vi "CTRE_Phoenix_CANcoder_GetPolymorphic.vi"   [LabVIEW 2020]
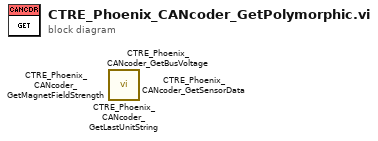
[diagram p0: block diagram]
diagram:
  n1 = call <vilib>:"CTRE_Phoenix_CANcoder_GetLastUnitString.vi"() -> ()  [unwired: 13 in, 3 out]
  n2 = call <vilib>:"CTRE_Phoenix_CANcoder_GetBusVoltage.vi"() -> ()  [unwired: 13 in, 3 out]
  n3 = call <vilib>:"CTRE_Phoenix_CANcoder_GetMagnetFieldStrength.vi"() -> ()  [unwired: 13 in, 3 out]
  n4 = call <vilib>:"CTRE_Phoenix_CANcoder_GetSensorData.vi"() -> ()  [unwired: 11 in, 5 out]
